vi "PAN_DBS_GetType.vi"(10 "cmd in":string, 11 "Database RefNum out":T1) -> (0 "datatype":string, 1 "value":string, 2 "name":string, 3 "value+dtype":string, 4 "precision":i32)   [LabVIEW 2016]
uses:
  Modules/DBSHAND/private/vis/DatabaseHand_RefNum.ctl
  Modules/DBSHAND/private/vis/DatabaseHand_Element_Get(I32).vi
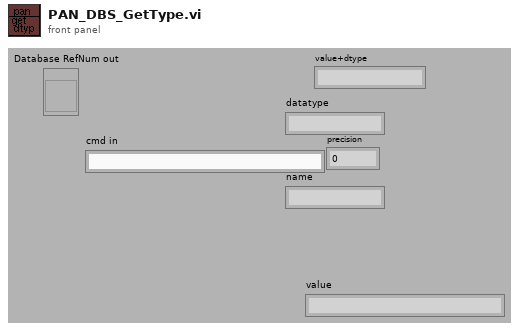
[diagram p1: front panel]
types:
  T1 = typedef "DatabaseHand_RefNum.ctl" = refnum<vi>
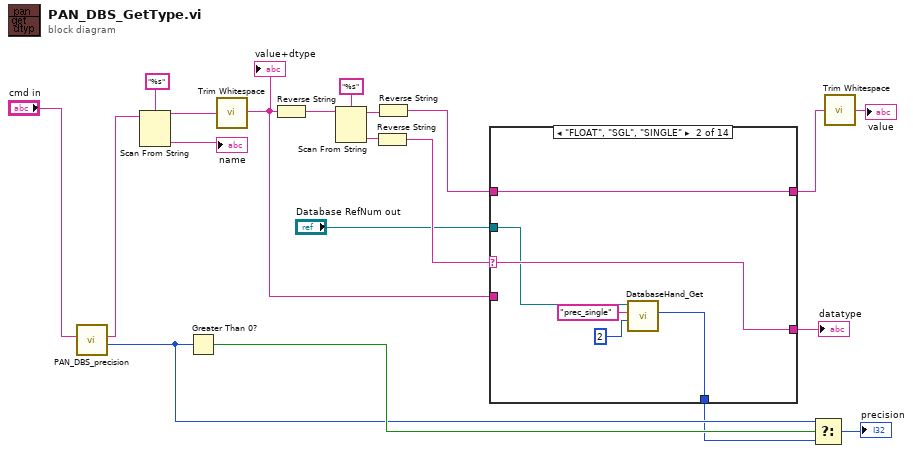
[diagram p0: block diagram]
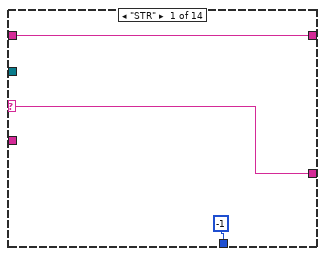
[diagram p2: hidden frame]
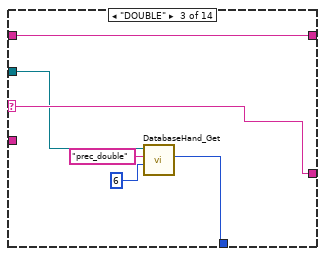
[diagram p3: hidden frame]
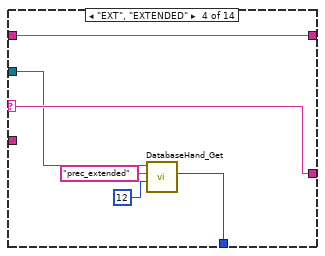
[diagram p4: hidden frame]
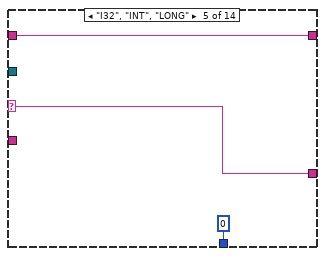
[diagram p5: hidden frame]
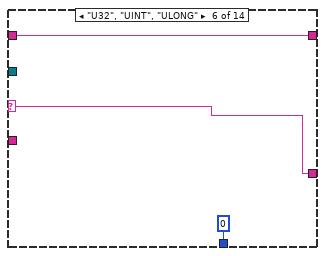
[diagram p6: hidden frame]
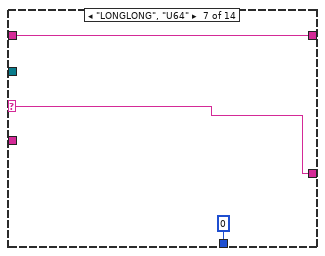
[diagram p7: hidden frame]
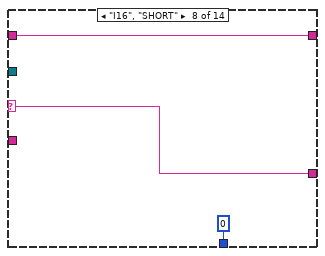
[diagram p8: hidden frame]
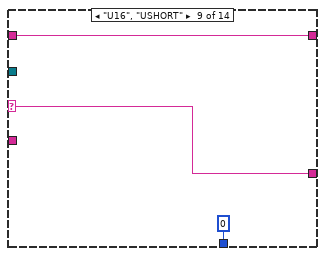
[diagram p9: hidden frame]
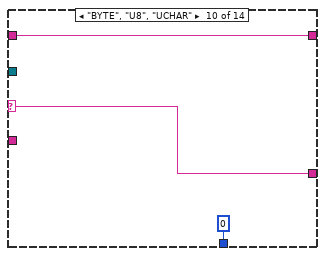
[diagram p10: hidden frame]
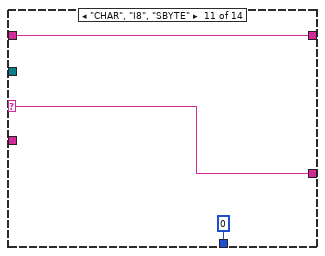
[diagram p11: hidden frame]
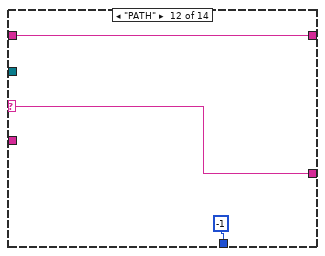
[diagram p12: hidden frame]
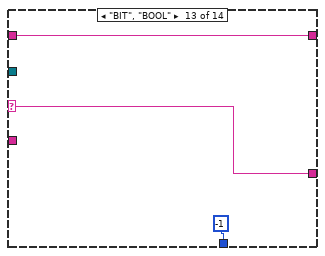
[diagram p13: hidden frame]
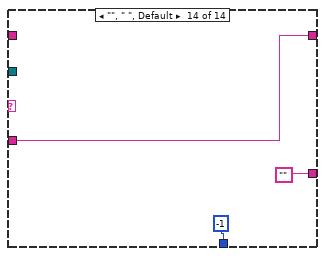
[diagram p14: hidden frame]
diagram:
  n1 = call "PAN_DBS_precision.vi"("args in"="cmd in") -> ("precision"=w3:i32, "args out"=w6:string)  [unwired: 9 out]
  n2 = Scan From String(format string="%s", input string=w6) -> (remaining string=w18:string, output 1=→"name":string)  [unwired: 2 in, 3 out]
  n3 = Greater Than 0?(x=w3) -> (x > 0?=w5:bool)
  n4 = call <vilib>:"Trim Whitespace.vi"("string"=w18) -> ("trimmed string"=w8:string)  [unwired: 1 in]
  "value+dtype" <- w8
  n5 = Reverse String(1:w8) -> (0:w17:string)
  n6 = Scan From String(format string="%s", input string=w17) -> (remaining string=w15:string, output 1=w13:string)  [unwired: 2 in, 3 out]
  n7 = Reverse String(1:w13) -> (0:w12:string)
  n8 = Reverse String(1:w15) -> (0:w10:string)
  n9 = case shown="\"FLOAT\", \"SGL\", \"SINGLE\"" w12 {
    selector: w12 -> [w23 w29 w35 w41 w44 w47 w50 w53 w56 w59 w62 w65 w68 _]
    tunnel: [w23 w29 w35 w41 w44 w47 w50 w53 w56 w59 w62 w65 w68 ""] -> w11
    tunnel: w10 -> [w22 w28 w34 w40 w43 w46 w49 w52 w55 w58 w61 w64 w67 _]
    tunnel: [w22 w28 w34 w40 w43 w46 w49 w52 w55 w58 w61 w64 w67 w70] -> w9
    tunnel: w8 -> [_ _ _ _ _ _ _ _ _ _ _ _ _ w70]
    tunnel: "Database RefNum out" -> [_ w25 w31 w39 _ _ _ _ _ _ _ _ _ _]
    tunnel: [-1 ("value") w24 w30 w36 0 ("value") 0 ("value") 0 ("value") 0 ("value") 0 ("value") 0 ("value") 0 ("value") -1 ("value") -1 ("value") -1 ("value")] -> w1
    frame "STR" {
    }
    frame "FLOAT", "SGL", "SINGLE" {
      n10 = call-poly "DatabaseHand_Get.vi"("default value"=2, "name"="prec_single", "Database RefNum in"=w25) -> ("value"=w24:i32)  [unwired: 2 in, 6 out]
    }
    frame "DOUBLE" {
      n11 = call-poly "DatabaseHand_Get.vi"("default value"=6, "name"="prec_double", "Database RefNum in"=w31) -> ("value"=w30:i32)  [unwired: 2 in, 6 out]
    }
    frame "EXT", "EXTENDED" {
      n12 = call-poly "DatabaseHand_Get.vi"("default value"=12, "name"="prec_extended", "Database RefNum in"=w39) -> ("value"=w36:i32)  [unwired: 2 in, 6 out]
    }
    frame "I32", "INT", "LONG" {
    }
    frame "U32", "UINT", "ULONG" {
    }
    frame "LONGLONG", "U64" {
    }
    frame "I16", "SHORT" {
    }
    frame "U16", "USHORT" {
    }
    frame "BYTE", "U8", "UCHAR" {
    }
    frame "CHAR", "I8", "SBYTE" {
    }
    frame "PATH" {
    }
    frame "BIT", "BOOL" {
    }
    frame "", " ", Default {
    }
  }
  "datatype" <- w11
  n13 = Select(t=w3, s=w5, f=w1) -> (s? t:f=→"precision":i32)
  n14 = call <vilib>:"Trim Whitespace.vi"("string"=w9) -> ("trimmed string"=→"value":string)  [unwired: 1 in]
